vi "Actor Core.vi"(8 "error in":errorcluster, 11 "SubPanel 3x3 View in":refnum<class "SubPanel 3x3 View.lvclass">) -> (0 "error out":errorcluster, 3 "Actor out":refnum<class "Actor.lvclass">)   [LabVIEW 2012, in "Win8uiDemo.lvlib" / "SubPanel 3x3 View.lvclass"]
doc: "(<B>Filename</B>: Actor Framework.lvlib:Actor.lvclass:Actor Core.vi)\n\nReceives messages to the actor, reacts to them, and initiates any error handling that may shut the actor down.\n\nDescendant classes may override this VI to append parallel tasks for the actor to complete while it handles messages. Overrides use the Call Parent Method node."
uses:
  SubPanel 3x3 View.lvclass
  <vilib>/ActorFramework/Actor/Actor.lvclass
  SubPanel Grid View.lvclass/SubPanel Grid View.ctl
  SubPanel Grid View.lvclass
  Write SubPanel Array.vi
  SubPanel Grid View/Write NextIndex.vi
  Win8uiFramework/ViewableActor.lvclass
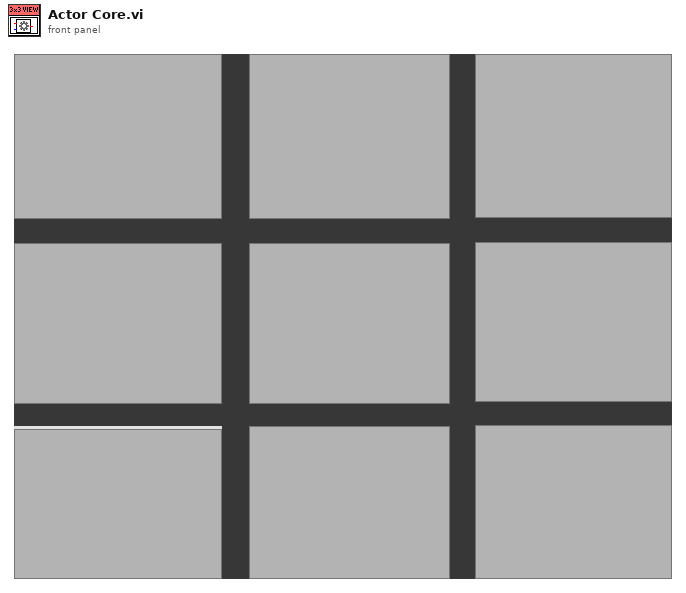
[diagram p1: front panel]
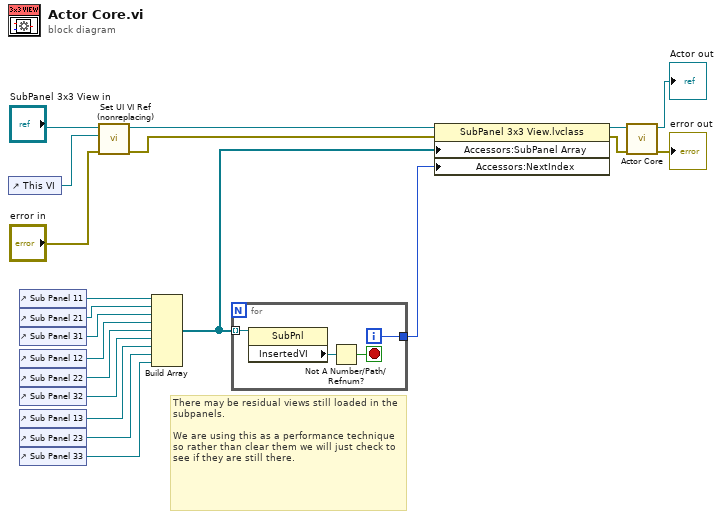
[diagram p0: block diagram]
diagram:
  # "There may be residual views still loaded in the subpanels.\n\nWe are using this as a performance technique so rather than clear them we will just check to see if they are still there."
  n1 = control-ref of="This VI"() -> (w16:refnum<vi>)
  n2 = control-ref of="Sub Panel 11"() -> (w14:refnum<vi>)
  n3 = control-ref of="Sub Panel 21"() -> (w13:refnum<vi>)
  n4 = control-ref of="Sub Panel 31"() -> (w12:refnum<vi>)
  n5 = control-ref of="Sub Panel 12"() -> (w11:refnum<vi>)
  n6 = control-ref of="Sub Panel 22"() -> (w10:refnum<vi>)
  n7 = control-ref of="Sub Panel 32"() -> (w9:refnum<vi>)
  n8 = control-ref of="Sub Panel 13"() -> (w8:refnum<vi>)
  n9 = control-ref of="Sub Panel 23"() -> (w7:refnum<vi>)
  n10 = control-ref of="Sub Panel 33"() -> (w6:refnum<vi>)
  n11 = call "Set UI VI Ref (nonreplacing).vi"("error in (no error)"="error in", "UI VI Ref"=w16, "ViewableActor in"="SubPanel 3x3 View in") -> ("error out"=w4:errorcluster, "ViewableActor out"=w18:refnum<class "SubPanel 3x3 View.lvclass">)  [unwired: 6 in, 1 out]
  n12 = Build Array(w14, w13, w12, w11, w10, w9, w8, w7, w6) -> (w2:refnum<vi>[])
  n13 = for {
    tunnel: w2 -> [w24] mode=indexing
    tunnel: [w21] -> w1
    i -> [w21]
    stop <- w22 stop-if-true
    n14 = property class="SubPnl"(reference=w24) -> ("InsertedVI"=w23:refnum<vi>)  [unwired: 1 in, 2 out]
    n15 = Not A Number/Path/Refnum?(number/path/refnum=w23) -> (NaN/Path/Refnum?=w22:bool)
  }
  n16 = property class="SubPanel 3x3 View.lvclass"(reference=w18, error in=w4, "Accessors:SubPanel Array"=w2, "Accessors:NextIndex"=w1) -> (reference out=w5:refnum<class "SubPanel 3x3 View.lvclass">, error out=w3:errorcluster)
  n17 = call-parent "Actor Core.vi"("error in"=w3, "MainView in"=w5) -> ("error out"=→"error out":errorcluster, "Actor out"=→"Actor out":refnum<class "Actor.lvclass">)  [unwired: 8 in]
